vi "Handle.vi"(11 "Base Event jettl in":refnum<class "Base Event jettl.lvclass">) -> (2 "Destroy?":bool, 3 "Base Event jettl out":refnum<class "Base Event jettl.lvclass">)   [LabVIEW 2021, in "jettl.lvlib" / "Base Event jettl.lvlib" / "Base Event jettl.lvclass"]
uses:
  Base Event jettl.lvclass
  C:/git/jettl/src/jettl/Actor/Event Actor/Event Actor.lvclass
  Base Event jettl.lvclass/Base Event jettl.ctl
  State/State/State.lvclass
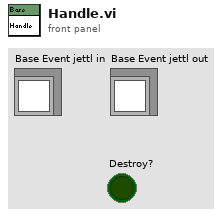
[diagram p1: front panel]
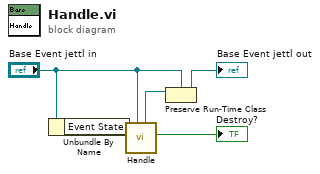
[diagram p0: block diagram]
diagram:
  n1 = Unbundle By Name("Base Event jettl in") -> ("Event State"=w4:refnum<class "State.lvclass">)
  n2 = call-dynamic "Handle.vi"("Event Actor in"="Base Event jettl in", "State in"=w4) -> ("Destroy?"=→"Destroy?":bool, "Event Actor out"=w2:refnum<class "Event Actor.lvclass">)  [unwired: 8 in]
  n3 = Preserve Run-Time Class(object in=w2, 2:"Base Event jettl in") -> (object out=→"Base Event jettl out":refnum<class "Base Event jettl.lvclass">)  [unwired: 1 in, 1 out]
